vi "Intake_Hopper_Pneumatic_Safety_Interlocks.vi"() -> (1 "Hopper Output":T1=enum."Reverse", 2 "Intake Output":T1=enum."Reverse")   [LabVIEW 2019]
uses:
  <vilib>/Rock Robotics/WPI/Solenoid/WPI_SolenoidValue.ctl
  Dashboard/CalibrationsGlobalVariables.vi
panel:
  out "Hopper Input":T1=enum."Reverse"
  out "Intake Input":T1=enum."Reverse"
  out "extend delay(ms)":dbl=1000.0
  out "retract delay(ms)":dbl=1000.0
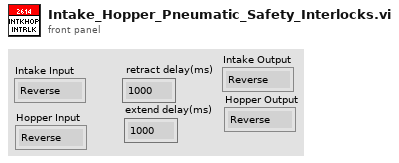
[diagram p1: front panel]
types:
  T1 = typedef "WPI_SolenoidValue.ctl" = enum16{"Off", "On", "Forward", "Reverse"}
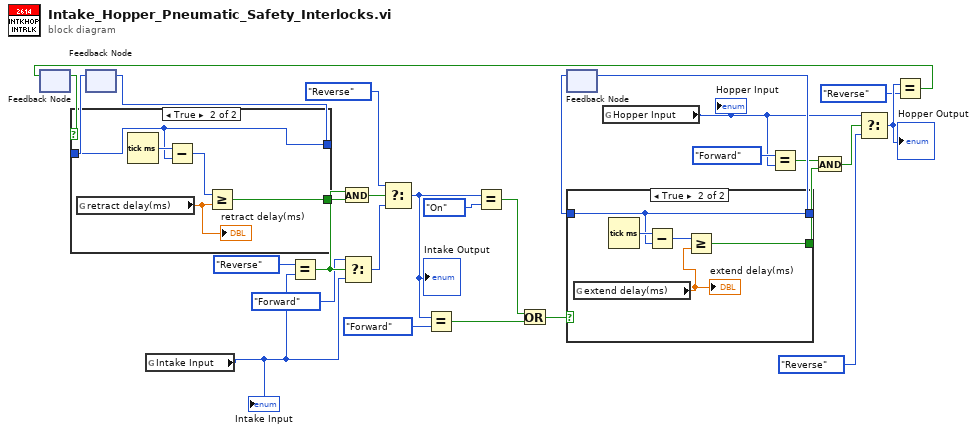
[diagram p0: block diagram]
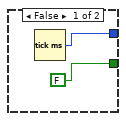
[diagram p2: hidden frame]
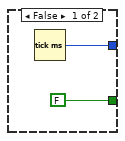
[diagram p3: hidden frame]
diagram:
  n1 = feedback #1() -> (w19:bool)  [unwired: 1 in]
  n2 = feedback #2() -> (w3:u32)  [unwired: 1 in]
  n3 = case shown="True" w19 {
    tunnel: [w29 w32] -> w4
    tunnel: [FALSE ("x .and. y?") w33] -> w20
    tunnel: w3 -> [_ w32]
    frame False {
      n4 = Tick Count (ms)() -> (millisecond timer value=w29:u32)
    }
    frame True {
      n5 = global read "CalibrationsGlobalVariables.vi" "retract delay(ms)"() -> (w31:dbl)
      "retract delay(ms)" <- w31
      n6 = Tick Count (ms)() -> (millisecond timer value=w35:u32)
      n7 = Subtract(x=w35, y=w32) -> (x-y=w34:u32)
      n8 = Greater Or Equal?(x=w34, y=w31) -> (x >= y?=w33:bool)
    }
  }
  n9 = feedback-in #2(w4) -> ()
  n10 = global read "CalibrationsGlobalVariables.vi" "Intake Input"() -> (w2:T1)
  "Intake Input" <- w2
  n11 = Equal?(x=WPI_SolenoidValue."Reverse" ("y"), y=w2) -> (x = y?=w21:bool)
  n12 = And(x=w21, y=w20) -> (x .and. y?=w22:bool)
  n13 = Select(t=WPI_SolenoidValue."Forward" ("y"), s=w21, f=w2) -> (s? t:f=w17:T1)
  n14 = Select(t=WPI_SolenoidValue."Reverse" ("y"), s=w22, f=w17) -> (s? t:f=w6:T1)
  "Intake Output" <- w6
  n15 = Equal?(x=w6, y=WPI_SolenoidValue."Forward") -> (x = y?=w9:bool)
  n16 = Equal?(x=w6, y=WPI_SolenoidValue."On") -> (x = y?=w10:bool)
  n17 = Or(x=w10, y=w9) -> (x .or. y?=w23:bool)
  n18 = feedback #3() -> (w28:u32)  [unwired: 1 in]
  n19 = case shown="True" w23 {
    tunnel: [w37 w39] -> w27
    tunnel: [FALSE ("x .and. y?") w40] -> w25
    tunnel: w28 -> [_ w39]
    frame False {
      n20 = Tick Count (ms)() -> (millisecond timer value=w37:u32)
    }
    frame True {
      n21 = global read "CalibrationsGlobalVariables.vi" "extend delay(ms)"() -> (w38:dbl)
      "extend delay(ms)" <- w38
      n22 = Tick Count (ms)() -> (millisecond timer value=w42:u32)
      n23 = Subtract(x=w42, y=w39) -> (x-y=w41:u32)
      n24 = Greater Or Equal?(x=w41, y=w38) -> (x >= y?=w40:bool)
    }
  }
  n25 = feedback-in #3(w27) -> ()
  n26 = global read "CalibrationsGlobalVariables.vi" "Hopper Input"() -> (w1:T1)
  "Hopper Input" <- w1
  n27 = Equal?(x=WPI_SolenoidValue."Forward" ("y"), y=w1) -> (x = y?=w26:bool)
  n28 = And(x=w26, y=w25) -> (x .and. y?=w24:bool)
  n29 = Select(t=w1, s=w24, f=WPI_SolenoidValue."Reverse" ("y")) -> (s? t:f=w13:T1)
  "Hopper Output" <- w13
  n30 = Equal?(x=w13, y=WPI_SolenoidValue."Reverse") -> (x = y?=w14:bool)
  n31 = feedback-in #1(w14) -> ()
